vi "Shutdown.vi"(8 "error in (no error)":errorcluster, 11 "Plugin Thread in":refnum<class "Plugin Thread.lvclass">) -> (0 "error out":errorcluster, 3 "Plugin Thread out":refnum<class "Plugin Thread.lvclass">)   [LabVIEW 2017, in "DSF Core.lvlib" / "Plugin Thread.lvclass"]
uses:
  Plugin Thread.lvclass
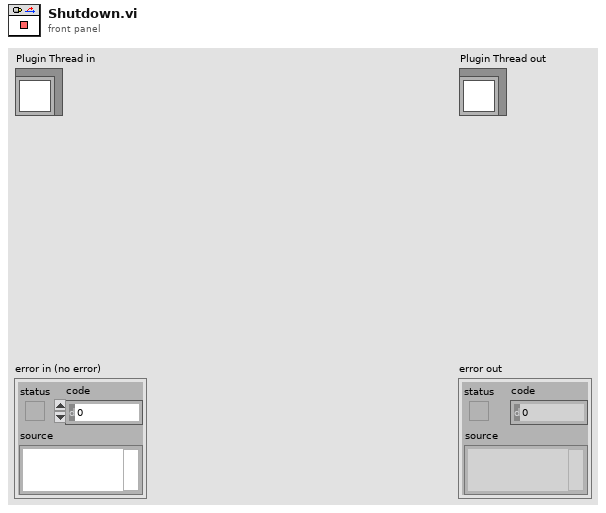
[diagram p1: front panel]
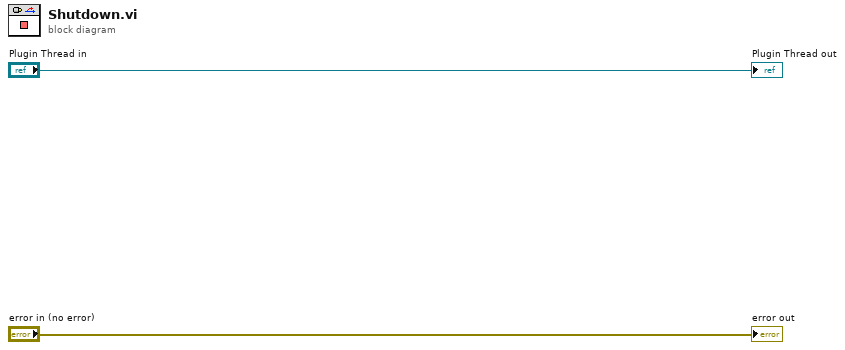
[diagram p0: block diagram]
diagram:
  "error out" <- "error in (no error)"
  "Plugin Thread out" <- "Plugin Thread in"
